vi "Construct.vi"(8 "error in (no error)":errorcluster, 11 "GUI Control Builder Director in":refnum<class "GUI Control Builder Director.lvclass">) -> (0 "error out":errorcluster, 2 "Panel Request Behavior":refnum<class "Panel Behavior.lvclass">, 3 "GUI Control Builder Director out":refnum<class "GUI Control Builder Director.lvclass">)   [LabVIEW 2015, in "GUI Control Builder Director.lvclass"]
uses:
  GUI Control Builder Director.lvclass
  _Depences/Panel API/Panel Request/Panle Requeset Behavior/Panel Behavior.lvclass
  GUI Control Builder Director.lvclass/GUI Control Builder Director.ctl
  GUI Controls/GUI Control/GUI Control.lvclass/GUI Control.ctl
  Control Builders/GUI Control Builder/GUI Control Builder.lvclass/GUI Control Builder.ctl
  Control Builders/GUI Control Builder/GUI Control Builder.lvclass
  GUI Controls/GUI Control/GUI Control.lvclass
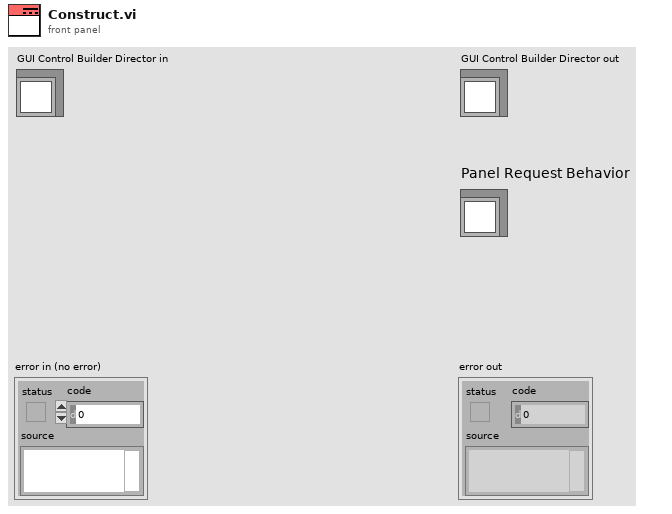
[diagram p1: front panel]
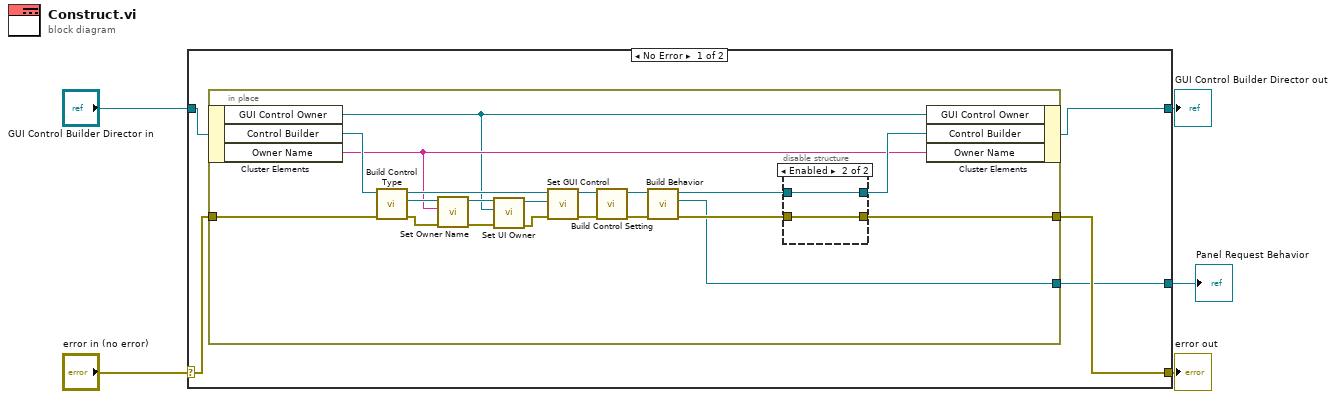
[diagram p0: block diagram]
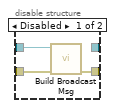
[diagram p2: hidden frame]
diagram:
  n1 = case shown="No Error" "error in (no error)" {
    selector: "error in (no error)" -> [w7 w37]
    tunnel: [w10 w37] -> w4
    tunnel: [w6 w36] -> w2
    tunnel: "GUI Control Builder Director in" -> [w8 w36]
    tunnel: [w9 _] -> w1
    frame No Error {
      n2 = in-place {
        in-place-border: [w23] -> w10
        in-place-border: [w22] -> w9
        in-place-border: w7 -> [w20]
        n3 = in-place-cluster #1(w8) -> ("GUI Control Owner"=w14:refnum<vi>, "Control Builder"=w21:refnum<class "GUI Control Builder.lvclass">, "Owner Name"=w16:string)
        n4 = call-dynamic "Build Control Type.vi"("error in (no error)"=w20, "Control Builder in"=w21) -> ("error out"=w17:errorcluster, "GUI Control"=w18:refnum<class "GUI Control.lvclass">, "Control Builder out"=w30:refnum<class "GUI Control Builder.lvclass">)  [unwired: 7 in]
        n5 = call "Set Owner Name.vi"("error in (no error)"=w17, "Owner Name"=w16, "GUI Control in"=w18) -> ("error out"=w13:errorcluster, "GUI Control out"=w15:refnum<class "GUI Control.lvclass">)  [unwired: 7 in]
        n6 = call "Set UI Owner.vi"("error in (no error)"=w13, "Owner"=w14, "GUI Control"=w15) -> ("error out"=w11:errorcluster, "GUI Control out"=w12:refnum<class "GUI Control.lvclass">)  [unwired: 7 in]
        n7 = call "Set GUI Control.vi"("error in (no error)"=w11, "GUI Control"=w12, "GUI Control Builder in"=w30) -> ("error out"=w28:errorcluster, "GUI Control Builder out"=w29:refnum<class "GUI Control Builder.lvclass">)  [unwired: 7 in]
        n8 = call "Build Control Setting.vi"("error in (no error)"=w28, "Control Builder in"=w29) -> ("error out"=w26:errorcluster, "Control Builder out"=w27:refnum<class "GUI Control Builder.lvclass">)  [unwired: 8 in]
        n9 = call-dynamic "Build Behavior.vi"("error in (no error)"=w26, "Control Builder in"=w27) -> ("error out"=w24:errorcluster, "Panel Request Behavior"=w22:refnum<class "Panel Behavior.lvclass">, "Control Builder out"=w25:refnum<class "GUI Control Builder.lvclass">)  [unwired: 7 in]
        n10 = disable-structure shown="Enabled" {
          disable-tunnel: w25 -> [w33 w34]
          disable-tunnel: w24 -> [w32 w35]
          disable-tunnel: [w31 w35] -> w23
          disable-tunnel: [_ w34] -> w19
          frame Disabled {
            n11 = call-dynamic "Build Broadcast Msg.vi"("error in (no error)"=w32, "Control Builder in"=w33) -> ("error out"=w31:errorcluster)  [unwired: 8 in, 1 out]
          }
          frame Enabled {
          }
        }
        n12 = in-place-cluster #1("GUI Control Owner"=w14, "Control Builder"=w19, "Owner Name"=w16) -> (w6:refnum<class "GUI Control Builder Director.lvclass">)
      }
    }
    frame Error {
    }
  }
  "error out" <- w4
  "GUI Control Builder Director out" <- w2
  "Panel Request Behavior" <- w1
